vi "Set Field Plot Cosmetics.vi"(8 "Position Estimation Method":u32(ring) items=["Star Configuration", "Swarm Method"], 9 "#Anchors":i32, 10 "#Tags":i32) -> (1 "Field Plot Cosmetics":T1(array[cluster]))   [LabVIEW 2014, in "Field.lvclass"]
doc: "This VI sets the proper field cosmetics for every plot in the field graph."
uses:
  Field.lvclass
panel:
  # "TODO: also do for swarm method"
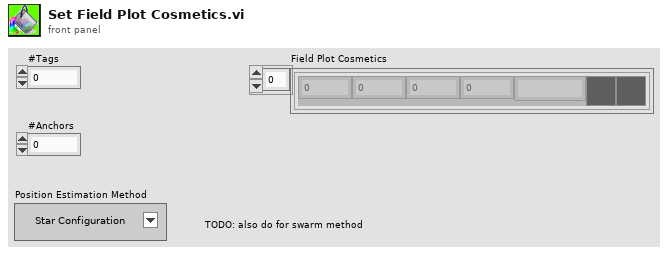
[diagram p1: front panel]
types:
  T1 = cluster{"Plot.Line Style":u8, "Plot.Line Width":u8, "Plot.Point Style":u8, "Plot.Plot Interpolation":u8, "Plot.Name":string, "Plot.Color":u32, "Fill / Point Color":u32}[]
  T2 = cluster{"Plot.Line Style":u8, "Plot.Line Width":u8, "Plot.Point Style":u8, "Plot.Plot Interpolation":u8, "Plot.Name":string, "Plot.Color":u32, "Plot.Fill/Point Color":u32}[]
  T3 = cluster{"Plot.Line Style":u8, "Plot.Line Width":u8, "Plot.Point Style":u8, "Plot.Plot Interpolation":u8, "String":string, "Color":u32, "Color":u32}
  T4 = cluster{"Plot.Line Style":u8, "Plot.Line Width":u8, "Plot.Point Style":u8, "Plot.Plot Interpolation":u8, "String":string, "Color":u32, "Color":u32}[]
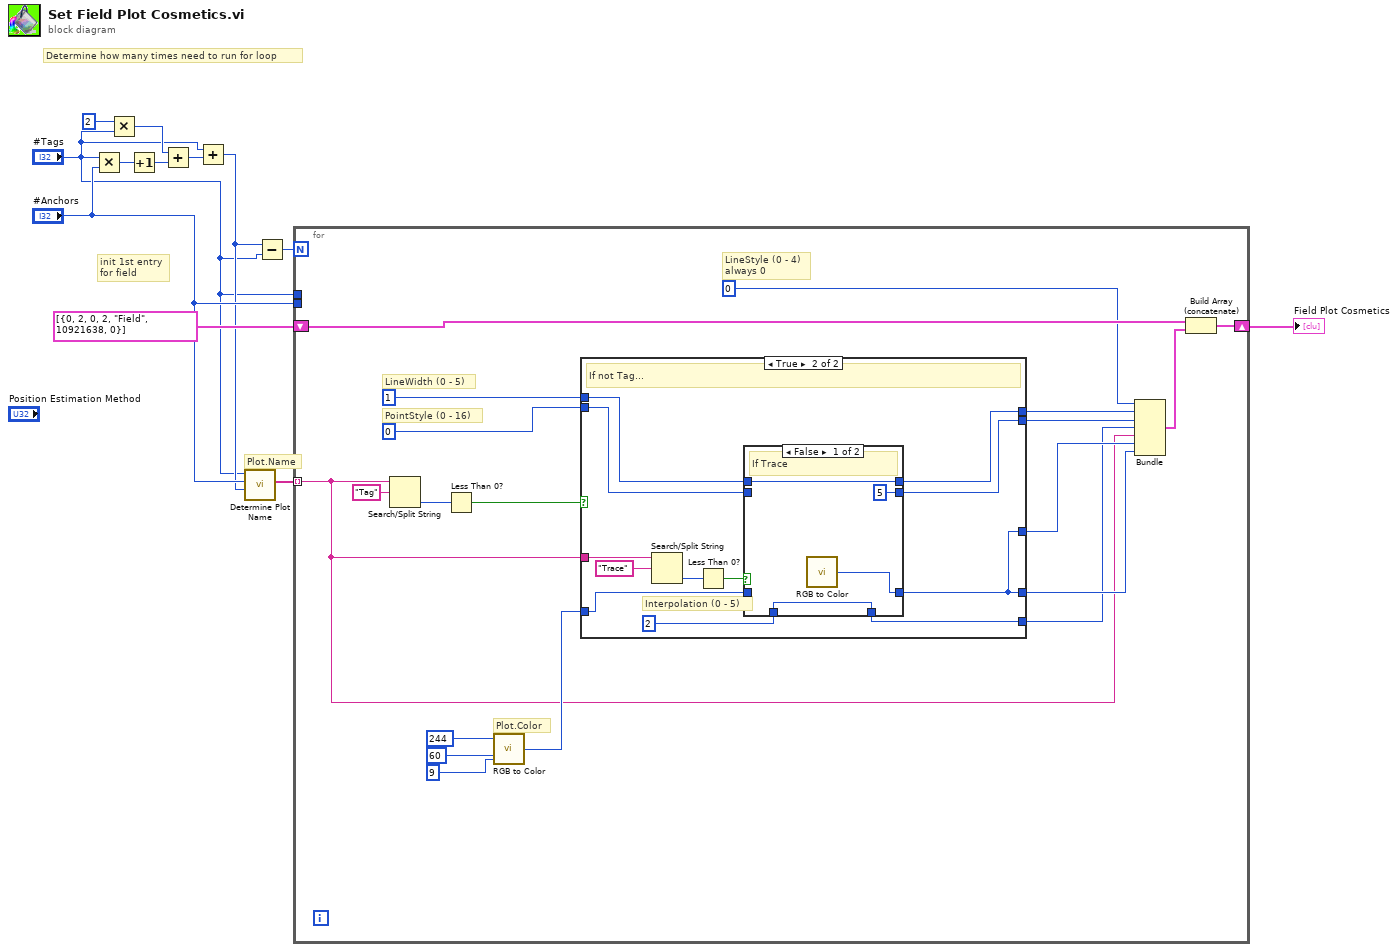
[diagram p0: block diagram]
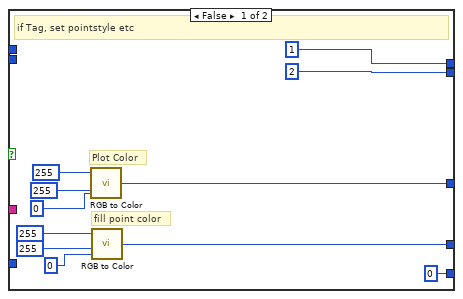
[diagram p2: hidden frame]
diagram:
  # "Plot.Name"
  # "init 1st entry\nfor field"
  # "Determine how many times need to run for loop"
  n1 = Multiply(x="#Tags", y="#Anchors") -> (x*y=w12:i32)
  n2 = Multiply(x=2, y="#Tags") -> (x*y=w9:i32)
  n3 = Increment(x=w12) -> (x+1=w11:i32)
  n4 = Add(x=w9, y=w11) -> (x+y=w8:i32)
  n5 = Add(x="#Tags", y=w8) -> (x+y=w2:i32)
  n6 = call "Determine Plot Name.vi"("n"=w2, "#anchors"="#Anchors", "#tags"="#Tags") -> ("Plot.Name Array"=w4:string[])  [unwired: 8 in]
  n7 = Subtract(x=w2, y="#Tags") -> (x-y=w3:i32)
  n8 = for {
    N: w3 -> [_]
    shift-right: [w28] -> w6
    shift-left: T2 [{"Plot.Line Style"=0, "Plot.Line Width"=2, "Plot.Point Style"=0, "Plot.Plot Interpolation"=2, "Plot.Name"="Field", "Plot.Color"=10921638, "Plot.Fill/Point Color"=0}] ("Field Plot Cosmetics") -> [w27]
    tunnel: "#Anchors" -> [_]
    tunnel: "#Tags" -> [_]
    tunnel: w4 -> [w14] mode=indexing
    # "PointStyle (0 - 16)"
    # "LineWidth (0 - 5)"
    # "LineStyle (0 - 4)\nalways 0"
    # "Plot.Color"
    n9 = Search/Split String(string=w14, search string/char (-)="Tag") -> (offset of match=w23:i32)  [unwired: 1 in, 2 out]
    n10 = Less Than 0?(x=w23) -> (x < 0?=w22:bool)
    n11 = call <vilib>:"RGB to Color.vi"("B"=u8 9, "G"=u8 60, "R"=u8 244) -> ("Color"=w17:u32)
    n12 = case shown="True" w22 {
      tunnel: u8 0 ("Plot.Point Style") -> [_ w50]
      tunnel: [u8 2 ("Plot.Point Style") w49] -> w20
      tunnel: u8 1 ("Plot.Line Width") -> [_ w46]
      tunnel: [u8 1 ("Plot.Line Width") w45] -> w18
      tunnel: w17 -> [_ w48]
      tunnel: [w38 w47] -> w16
      tunnel: [w36 w47] -> w15
      tunnel: w14 -> [_ w53]
      tunnel: [u8 0 ("Plot.Plot Interpolation") w43] -> w13
      frame False {
        # "fill point color"
        # "Plot Color"
        # "if Tag, set pointstyle etc"
        n13 = call <vilib>:"RGB to Color.vi"("B"=u8 0, "G"=u8 255, "R"=u8 255) -> ("Color"=w38:u32)
        n14 = call <vilib>:"RGB to Color.vi"("B"=u8 0, "G"=u8 255, "R"=u8 255) -> ("Color"=w36:u32)
      }
      frame True {
        # "Interpolation (0 - 5)"
        # "If not Tag..."
        n15 = Search/Split String(string=w53, search string/char (-)="Trace" ("string")) -> (offset of match=w52:i32)  [unwired: 1 in, 2 out]
        n16 = Less Than 0?(x=w52) -> (x < 0?=w51:bool)
        n17 = case shown="False" w51 {
          tunnel: w50 -> [_ w62]
          tunnel: [u8 5 ("Plot.Point Style") w62] -> w49
          tunnel: w48 -> [_ w61]
          tunnel: [w56 w61] -> w47
          tunnel: w46 -> [w58 w60]
          tunnel: [w58 w60] -> w45
          tunnel: u8 2 ("Plot.Plot Interpolation") -> [w55 w59]
          tunnel: [w55 w59] -> w43
          frame False {
            # "If Trace"
            n18 = call <vilib>:"RGB to Color.vi"() -> ("Color"=w56:u32)  [unwired: 3 in]
          }
          frame True {
            # "If Anchor"
          }
        }
      }
    }
    n19 = Bundle("Plot.Line Style"=u8 0, "Plot.Line Width"=w18, "Plot.Point Style"=w20, "Plot.Plot Interpolation"=w13, "String"=w14, "Color"=w16, "Color"=w15) -> (w25:T3)  [unwired: 1 in]
    n20 = Build Array (concatenate)(w27, w25) -> (w28:T4)
  }
  "Field Plot Cosmetics" <- w6
